vi "Infeed_Pneumatics.vi"(9 "Eject":bool, 10 "Station":bool, 11 "Floor":bool) -> (3 "Boolean":bool)   [LabVIEW 2014]
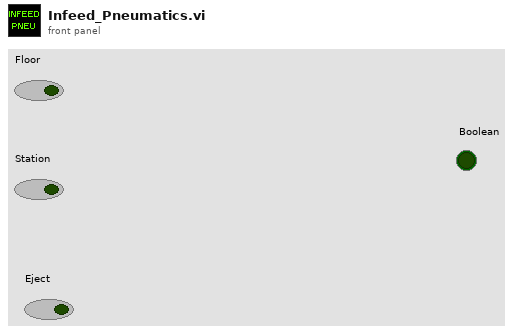
[diagram p1: front panel]
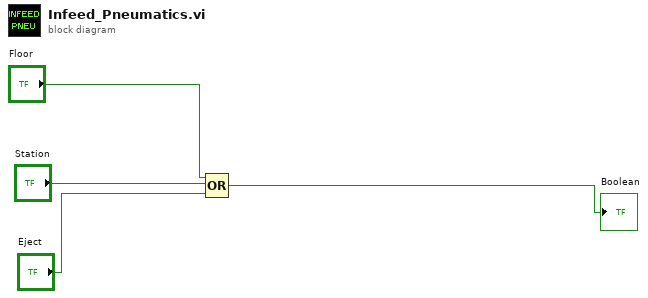
[diagram p0: block diagram]
diagram:
  n1 = Compound Arithmetic op=OR("Floor", "Station", "Eject") -> (→"Boolean":bool)
